vi "H5Lget_name_by_idx.vi"(5 "Order":T1 items=["H5_ITER_UNKNOWN"=-1, "H5_ITER_INC"=0, "H5_ITER_DEC"=1], 6 "lapl_id":T3, 7 "Index Field":T2 items=["H5_INDEX_UNKNOWN"=-1, "H5_INDEX_NAME"=0, "H5_INDEX_CRT_ORDER"=1], 8 "error in (no error)":errorcluster, 9 "Index":u64, 10 "Group Name":string=".", 11 "Location Ref":T3) -> (0 "error out":errorcluster, 2 "Item Name":string, 3 "Location Ref out":T3)   [LabVIEW 2017]
doc: "Retrieves name of the nth link in a group, \n according to the order within a specified field or index."
uses:
  <vilib>/UPVI/lvhdf5/library.llb/HDF5 Ref.ctl
  <vilib>/UPVI/lvhdf5/library.llb/H5_index_t.ctl
  <vilib>/UPVI/lvhdf5/library.llb/H5_iter_order_t.ctl
  <vilib>/UPVI/lvhdf5/hdf5.dll
panel:
  # "LVHDF5 Toolkit\nCopyright (c) 2005-2013 by Jason D. Sommerville\nCopyright (c) 2014-2015 by UPVI, LLC.\n\nThis use and distribution of this file is governed by the terms found in \nLICENSE.txt distributed with this toolkit and installed at\n <user.lib>\\_lvhdf5\\LICENSE.txt"
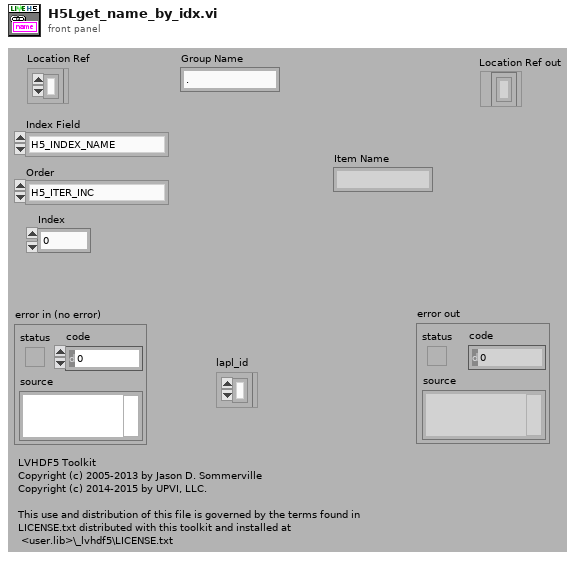
[diagram p1: front panel]
types:
  T1 = typedef "H5_iter_order_t.ctl" = i32
  T2 = typedef "H5_index_t.ctl" = i32
  T3 = typedef "HDF5 Ref.ctl" = refnum<k1>
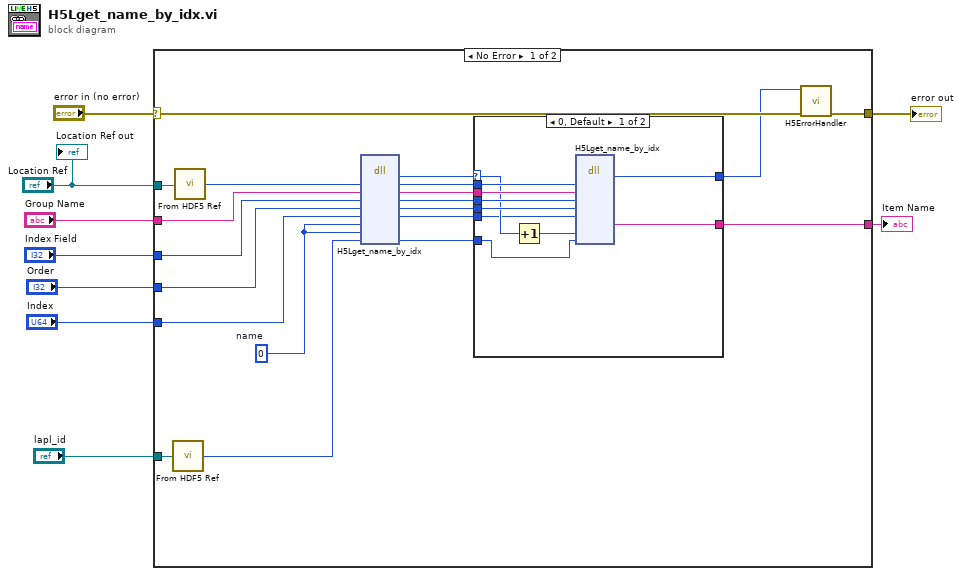
[diagram p0: block diagram]
diagram:
  n1 = case shown="No Error" "error in (no error)" {
    selector: "error in (no error)" -> [w29 w41]
    tunnel: [w28 w41] -> w8
    tunnel: "lapl_id" -> [w27 _]
    tunnel: "Location Ref" -> [w25 _]
    tunnel: "Group Name" -> [w23 _]
    tunnel: "Index Field" -> [w22 _]
    tunnel: "Order" -> [w21 _]
    tunnel: "Index" -> [w20 _]
    tunnel: [w11 _] -> w1
    frame No Error {
      w13 = u64 0  # name
      n2 = call <vilib>:"From HDF5 Ref.vi"("HDF5 Ref"=w27) -> ("I32"=w26:i32)
      n3 = call <vilib>:"From HDF5 Ref.vi"("HDF5 Ref"=w25) -> ("I32"=w24:i32)
      n4 = dll-call lib="C:/Program Files/National Instruments/LabVIEW 2017/vi.lib/UPVI/lvhdf5/hdf5.dll" fn="H5Lget_name_by_idx"("loc_id"=w24, "group_name"=w23, "index_field"=w22, "order"=w21, "n"=w20, "name"=w13, "size"=w13, "lapl_id"=w26) -> ("return type"=w19:i32, "loc_id"=w17:i32, "group_name"=w16:string, "index_field"=w15:i32, "order"=w14:i32, "n"=w10:u64, "lapl_id"=w12:i32)  [unwired: 5 in, 2 out]
      n5 = case shown="0, Default" w19 {
        selector: w19 -> [w35 w40]
        tunnel: [w31 w40] -> w18
        tunnel: w17 -> [w39 _]
        tunnel: w16 -> [w38 _]
        tunnel: w15 -> [w37 _]
        tunnel: w14 -> [w36 _]
        tunnel: w12 -> [w33 _]
        tunnel: [w32 _] -> w11
        tunnel: w10 -> [w30 _]
        frame 0, Default {
          n6 = Increment(x=w35) -> (x+1=w34:i32)
          n7 = dll-call lib="C:/Program Files/National Instruments/LabVIEW 2017/vi.lib/UPVI/lvhdf5/hdf5.dll" fn="H5Lget_name_by_idx"("loc_id"=w39, "group_name"=w38, "index_field"=w37, "order"=w36, "n"=w30, "size"=w34, "lapl_id"=w33) -> ("return type"=w31:i32, "name"=w32:string)  [unwired: 11 in, 2 out]
        }
        frame -1 {
        }
      }
      n8 = call <vilib>:"H5ErrorHandler.vi"("error in (no error)"=w29, "herr_t"=w18) -> ("error out"=w28:errorcluster)  [unwired: 3 in, 4 out]
    }
    frame Error {
    }
  }
  "error out" <- w8
  "Item Name" <- w1
  "Location Ref out" <- "Location Ref"
